vi "AB_Apply_RESTful_VI_Configuration.vi"(8 "error in (no error)":errorcluster, 10 "RESTful VI configuration":T1={"Service VI Type"=enum."Web Method", "Load VI at statup"=TRUE, "Keep VI in memory"=TRUE, "Output type"=enum."Terminal", "Output format"=enum."XML", "Use headers"=TRUE, "Buffered"=TRUE, "eng_Load VI by name"=FALSE}, 11 "VI in":refnum<class "AB_Source_VI.lvclass">) -> (0 "error out":errorcluster, 3 "VI out":refnum<class "AB_Source_VI.lvclass">)   [LabVIEW 2020]
uses:
  <vilib>/AppBuilder/AB_Classes/Source/VI/AB_Source_VI.lvclass
  <vilib>/AppBuilder/AB_Classes/Source/RESTfulVI/Configure_RESTfulVI/AB_RESTful_Configuration.ctl
  <vilib>/AppBuilder/AB_Classes/Source/RESTfulVI/Configure_RESTfulVI/AB_RESTful_VIType.ctl
  <vilib>/AppBuilder/AB_Classes/Source/RESTfulVI/Configure_RESTfulVI/AB_RESTful_OutputType.ctl
  <vilib>/AppBuilder/AB_Classes/Source/RESTfulVI/Configure_RESTfulVI/AB_RESTful_OutputFormat.ctl
  <vilib>/AppBuilder/AB_Classes/Source/RESTfulVI/AB_Source_RESTfulVI.lvclass
  e:/builds/penguin/labview/branches/2020/dev/dist/vi.lib/AppBuilder/AB_Classes/Source/VI/AB_Source_VI.lvclass
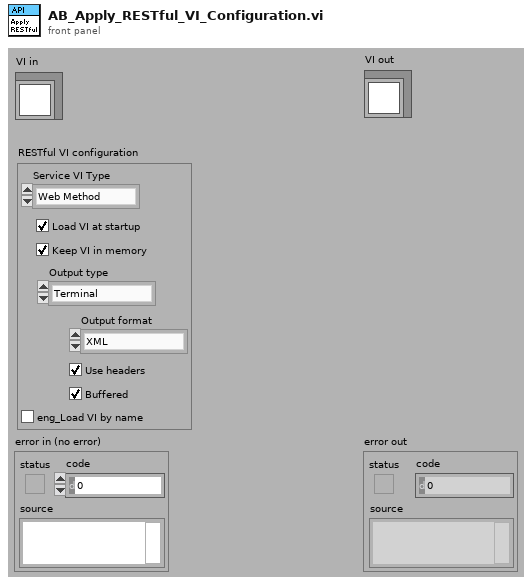
[diagram p1: front panel]
types:
  T1 = typedef "AB_RESTful_Configuration.ctl" = cluster{"Service VI Type":T2, "Load VI at statup":bool, "Keep VI in memory":bool, "Output type":T3, "Output format":T4, "Use headers":bool, "Buffered":bool, "eng_Load VI by name":bool}
  T2 = typedef "AB_RESTful_VIType.ctl" = enum32{"Web Method", "Auxiliary", "eng_Internal", "eng_Content"}
  T3 = typedef "AB_RESTful_OutputType.ctl" = enum32{"Terminal", "Stream"}
  T4 = typedef "AB_RESTful_OutputFormat.ctl" = enum32{"XML", "Text", "HTML", "JSON"}
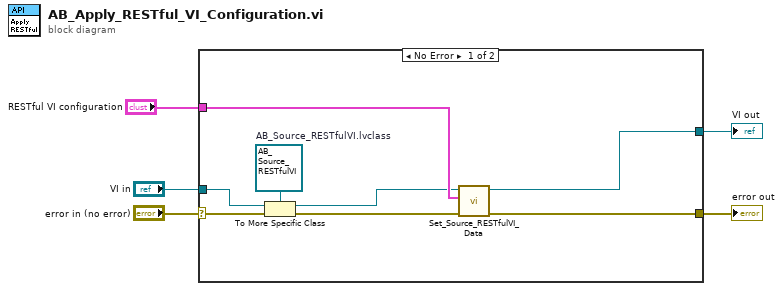
[diagram p0: block diagram]
diagram:
  n1 = case shown="No Error" "error in (no error)" {
    selector: "error in (no error)" -> [w12 w14]
    tunnel: [w7 w14] -> w4
    tunnel: "VI in" -> [w13 _]
    tunnel: [w6 _] -> w2
    tunnel: "RESTful VI configuration" -> [w10 _]
    frame No Error {
      w11 = refnum<class "AB_Source_RESTfulVI.lvclass"> refnum  # AB_Source_RESTfulVI.lvclass
      n2 = To More Specific Class(target class=w11, reference=w13, error in=w12) -> (specific class reference=w9:refnum<class "AB_Source_RESTfulVI.lvclass">, error out=w8:errorcluster)
      n3 = call <vilib>:"Set_Source_RESTfulVI_Data.vi"("error in (no error)"=w8, "RESTful VI configuration"=w10, "Class in"=w9) -> ("error out"=w7:errorcluster, "Class out"=w6:refnum<class "AB_Source_RESTfulVI.lvclass">)  [unwired: 7 in]
    }
    frame Error {
    }
  }
  "error out" <- w4
  "VI out" <- w2
